vi "Main.vi"(8 "error in (no error)":errorcluster, 11 "RSABase in":refnum<class "RSA.lvclass">) -> (0 "error out":errorcluster, 3 "component":refnum<class "RSA.lvclass">)   [LabVIEW 2012, in "RSA.lvclass"]
doc: "Main VI of the component."
uses:
  RSA.lvclass
  <vilib>/Distrio/Murmex/Murmex/command_enum.ctl
  starting shape.ctl
  RSA.lvclass/RSA.ctl
  <vilib>/Distrio/Murmex/InitialiseMessage/InitialiseMessage.lvclass
  <vilib>/Distrio/Murmex/TerminateMessage/TerminateMessage.lvclass
  <vilib>/Distrio/Murmex/ConfigureMessage/ConfigureMessage.lvclass
  <vilib>/Distrio/Murmex/StartMessage/StartMessage.lvclass
  <vilib>/Distrio/Murmex/Murmex/update_cluster.ctl
  <vilib>/Distrio/Murmex/ResetMessage/ResetMessage.lvclass
  <vilib>/Distrio/Murmex/Murmex/Set configure at initialise.vi
  <vilib>/Distrio/Murmex/Murmex/Set log reference.vi
  <vilib>/Distrio/Murmex/Murmex/Set VI reference.vi
  <vilib>/Distrio/Murmex/Murmex/Get ID.vi
  <vilib>/Distrio/Murmex/Murmex/Murmex.lvclass
  <vilib>/Distrio/Murmex/Message/Message.lvclass
panel:
  in  "button::stop":bool
  in  "button::reset":bool
  in  "button::start":bool
  in  "button::quit":bool
  in  "Tab Control":enum32{"Settings", "Indicators", "Debug"}(tab)
  in  "Starting shape":T1
  in  "Bunch for averaging":i32=12
  in  "Wait time [ms]":u32=50
  in  "stop after":i32=500
  in  "Iterations until BC":i32=5000
  in  "Search Range [%]":dbl(knob)=100.0 min=0.0 max=100.0 step=5.0 scale=0.0..100.0
  in  "Optimisation name":string="bob"
  out "current MF":cluster{"Y":dbl[], "Y":dbl[]}[](graph)
  out "unsuccessfull iterations":i32
  out "successfull iterations":i32
  out "current Merit Factor":dbl
  out "Iterations since last improvement":i32
  out "max Merit Factor":dbl
  out "BC on":bool
  out "MF standard deviation":dbl
  out "best MF":cluster{"Y":dbl[], "Y":dbl[]}[](graph)
  out "BC counter":i32
  out "log":string="\r\n11:11:41.970 05/12/2013: initialise from AOTF to AOTF\r\n11:11:42.586 05/12/2013: inform from AOTF to AOTF\r\n11:11:43.913 05/12/2013: update from AOTF to AOTF\r\n11:11:45.142 05/12/2013: generic (shutter_off) from AOTF to AOTF\r\n11:11:45.270 05/12/2013: generic (shutter_on) from AOTF to AOTF\r\n11:11:45.902 05/12/2013: generic (shutter_off) from AOTF to AOTF\r\n11:11:45.932 05/12/2013: inspect from AOTF to AOTF\r\n11:11:48.013 05/12/2013: configure from AOTF to AOTF\r\n11:11:52.003 05/12/2013: inform from AOTF to AOTF\r\n11:11:58.521 05/12/2013: initialise from AOTF to AOTF\r\n11:11:58.561 05/12/2013: inform from AOTF to AOTF\r\n11:11:58.695 05/12/2013: inform from AOTF to AOTF\r\n11:12:02.089 05/12/2013: update from AOTF to AOTF\r\n11:12:02.308 05/12/2013: inspect from AOTF to AOTF\r\n11:12:02.364 05/12/2013: inform from AOTF to AOTF\r\n11:12:05.062 05/12/2013: generic (shutter_on) from AOTF to AOTF\r\n11:12:06.690 05/12/2013: update from AOTF to AOTF\r\n11:12:06.909 05/12/2013: inspect from AOTF to AOTF\r\n11:12:06.964 05/12/2013: inform from AOTF to AOTF\r\n11:12:07.770 05/12/2013: update from AOTF to AOTF\r\n11:12:07.989 05/12/2013: inspect from AOTF to AOTF\r\n11:12:08.044 05/12/2013: inform from AOTF to AOTF\r\n11:12:08.627 05/12/2013: update from AOTF to AOTF\r\n11:12:08.846 05/12/2013: inspect from AOTF to AOTF\r\n11:12:08.900 05/12/2013: inform from AOTF to AOTF\r\n11:12:09.290 05/12/2013: update from AOTF to AOTF\r\n11:12:09.508 05/12/2013: inspect from AOTF to AOTF\r\n11:12:09.563 05/12/2013: inform from AOTF to AOTF\r\n11:12:10.154 05/12/2013: update from AOTF to AOTF\r\n11:12:10.373 05/12/2013: inspect from AOTF to AOTF\r\n11:12:10.430 05/12/2013: inform from AOTF to AOTF\r\n11:12:20.953 05/12/2013: update from AOTF to AOTF\r\n11:12:21.172 05/12/2013: inspect from AOTF to AOTF\r\n11:12:21.227 05/12/2013: inform from AOTF to AOTF\r\n11:12:22.057 05/12/2013: update from AOTF to AOTF\r\n11:12:22.276 05/12/2013: inspect from AOTF to AOTF\r\n11:12:22.330 05/12/2013: inform from AOTF to AOTF\r\n11:12:22.841 05/12/2013: update from AOTF to AOTF\r\n11:12:23.060 05/12/2013: inspect from AOTF to AOTF\r\n11:12:23.114 05/12/2013: inform from AOTF to AOTF\r\n11:12:23.449 05/12/2013: update from AOTF to AOTF\r\n11:12:23.668 05/12/2013: inspect from AOTF to AOTF\r\n11:12:23.724 05/12/2013: inform from AOTF to AOTF\r\n11:12:24.514 05/12/2013: update from AOTF to AOTF\r\n11:12:24.733 05/12/2013: inspect from AOTF to AOTF\r\n11:12:24.789 05/12/2013: inform from AOTF to AOTF\r\n11:12:25.098 05/12/2013: update from AOTF to AOTF\r\n11:12:25.317 05/12/2013: inspect from AOTF to AOTF\r\n11:12:25.371 05/12/2013: inform from AOTF to AOTF\r\n11:12:26.482 05/12/2013: update from AOTF to AOTF\r\n11:12:26.701 05/12/2013: inspect from AOTF to AOTF\r\n11:12:26.755 05/12/2013: inform from AOTF to AOTF\r\n11:12:27.154 05/12/2013: update from AOTF to AOTF\r\n11:12:27.373 05/12/2013: inspect from AOTF to AOTF\r\n11:12:27.428 05/12/2013: inform from AOTF to AOTF\r\n11:12:27.666 05/12/2013: update from AOTF to AOTF\r\n11:12:27.885 05/12/2013: inspect from AOTF to AOTF\r\n11:12:27.944 05/12/2013: inform from AOTF to AOTF\r\n11:12:33.380 05/12/2013: update from AOTF to AOTF\r\n11:12:33.484 05/12/2013: update from AOTF to AOTF\r\n11:12:33.603 05/12/2013: inspect from AOTF to AOTF\r\n11:12:33.611 05/12/2013: update from AOTF to AOTF\r\n11:12:33.684 05/12/2013: update from AOTF to AOTF\r\n11:12:33.740 05/12/2013: update from AOTF to AOTF\r\n11:12:33.827 05/12/2013: inspect from AOTF to AOTF\r\n11:12:33.835 05/12/2013: update from AOTF to AOTF\r\n11:12:33.897 05/12/2013: inform from AOTF to AOTF\r\n11:12:33.903 05/12/2013: update from AOTF to AOTF\r\n11:12:33.940 05/12/2013: update from AOTF to AOTF\r\n11:12:34.085 05/12/2013: update from AOTF to AOTF\r\n11:12:34.119 05/12/2013: inspect from AOTF to AOTF\r\n11:12:34.292 05/12/2013: update from AOTF to AOTF\r\n11:12:34.336 05/12/2013: inspect from AOTF to AOTF\r\n11:12:34.553 05/12/2013: inspect from AOTF to AOTF\r\n11:12:34.608 05/12/2013: inform from AOTF to AOTF\r\n11:12:34.739 05/12/2013: update from AOTF to AOTF\r\n11:12:34.771 05/12/2013: update from AOTF to AOTF\r\n11:12:34.826 05/12/2013: inspect from AOTF to AOTF\r\n11:12:34.834 05/12/2013: update from AOTF to AOTF\r\n11:12:34.867 05/12/2013: update from AOTF to AOTF\r\n11:12:34.931 05/12/2013: update from AOTF to AOTF\r\n11:12:34.979 05/12/2013: update from AOTF to AOTF\r\n11:12:35.003 05/12/2013: update from AOTF to AOTF\r\n11:12:35.027 05/12/2013: update from AOTF to AOTF\r\n11:12:35.041 05/12/2013: update from AOTF to AOTF\r\n11:12:35.051 05/12/2013: inspect from AOTF to AOTF\r\n11:12:35.066 05/12/2013: update from AOTF to AOTF\r\n11:12:35.116 05/12/2013: update from AOTF to AOTF\r\n11:12:35.171 05/12/2013: update from AOTF to AOTF\r\n11:12:35.211 05/12/2013: update from AOTF to AOTF\r\n11:12:35.273 05/12/2013: inspect from AOTF to AOTF\r\n11:12:35.287 05/12/2013: update from AOTF to AOTF\r\n11:12:35.475 05/12/2013: update from AOTF to AOTF\r\n11:12:35.495 05/12/2013: inspect from AOTF to AOTF\r\n11:12:35.549 05/12/2013: inform from AOTF to AOTF\r\n11:12:35.764 05/12/2013: inspect from AOTF to AOTF\r\n11:12:35.819 05/12/2013: inform from AOTF to AOTF\r\n11:12:35.861 05/12/2013: update from AOTF to AOTF\r\n11:12:35.877 05/12/2013: inform from AOTF to AOTF\r\n11:12:35.947 05/12/2013: update from AOTF to AOTF\r\n11:12:36.067 05/12/2013: update from AOTF to AOTF\r\n11:12:36.100 05/12/2013: inspect from AOTF to AOTF\r\n11:12:36.235 05/12/2013: update from AOTF to AOTF\r\n11:12:36.317 05/12/2013: inspect from AOTF to AOTF\r\n11:12:36.371 05/12/2013: inform from AOTF to AOTF\r\n11:12:36.587 05/12/2013: inspect from AOTF to AOTF\r\n11:12:36.771 05/12/2013: update from AOTF to AOTF\r\n11:12:36.804 05/12/2013: inspect from AOTF to AOTF\r\n11:12:37.020 05/12/2013: inspect from AOTF to AOTF\r\n11:12:37.238 05/12/2013: inspect from AOTF to AOTF\r\n11:12:37.456 05/12/2013: inspect from AOTF to AOTF\r\n11:12:37.673 05/12/2013: inspect from AOTF to AOTF\r\n11:12:37.891 05/12/2013: inspect from AOTF to AOTF\r\n11:12:37.946 05/12/2013: inform from AOTF to AOTF\r\n11:12:38.161 05/12/2013: inspect from AOTF to AOTF\r\n11:12:38.379 05/12/2013: inspect from AOTF to AOTF\r\n11:12:38.597 05/12/2013: inspect from AOTF to AOTF\r\n11:12:38.815 05/12/2013: inspect from AOTF to AOTF\r\n11:12:38.871 05/12/2013: inform from AOTF to AOTF\r\n11:12:39.086 05/12/2013: inspect from AOTF to AOTF\r\n11:12:39.303 05/12/2013: inspect from AOTF to AOTF\r\n11:12:39.363 05/12/2013: inform from AOTF to AOTF\r\n11:12:39.417 05/12/2013: inform from AOTF to AOTF\r\n11:12:39.633 05/12/2013: inspect from AOTF to AOTF\r\n11:12:39.852 05/12/2013: inspect from AOTF to AOTF\r\n11:12:40.069 05/12/2013: inspect from AOTF to AOTF\r\n11:12:40.124 05/12/2013: inform from AOTF to AOTF\r\n11:12:40.339 05/12/2013: inspect from AOTF to AOTF\r\n11:12:40.395 05/12/2013: inform from AOTF to AOTF\r\n11:12:40.448 05/12/2013: inform from AOTF to AOTF\r\n11:12:40.663 05/12/2013: inspect from AOTF to AOTF\r\n11:12:40.718 05/12/2013: inform from AOTF to AOTF\r\n11:12:40.770 05/12/2013: inform from AOTF to AOTF\r\n11:12:40.824 05/12/2013: inform from AOTF to AOTF\r\n11:12:40.877 05/12/2013: inform from AOTF to AOTF\r\n11:12:40.930 05/12/2013: inform from AOTF to AOTF\r\n11:12:40.982 05/12/2013: inform from AOTF to AOTF\r\n11:12:41.034 05/12/2013: inform from AOTF to AOTF\r\n11:12:41.092 05/12/2013: inform from AOTF to AOTF\r\n11:12:41.144 05/12/2013: inform from AOTF to AOTF\r\n11:12:41.196 05/12/2013: inform from AOTF to AOTF\r\n11:12:41.249 05/12/2013: inform from AOTF to AOTF\r\n11:12:41.307 05/12/2013: inform from AOTF to AOTF\r\n11:12:41.366 05/12/2013: inform from AOTF to AOTF\r\n11:12:41.424 05/12/2013: inform from AOTF to AOTF\r\n11:12:41.478 05/12/2013: inform from AOTF to AOTF\r\n11:12:41.533 05/12/2013: inform from AOTF to AOTF\r\n11:12:41.589 05/12/2013: inform from AOTF to AOTF\r\n11:12:42.246 05/12/2013: terminate from AOTF to AOTF"
  in  "component ID":string="RSA"
  in  "command":T2
  in  "Generic command":string
  in  "button::configure":bool
  in  "button::send":bool
  out "terminate?":bool=TRUE
  # "RSA settings"
  # "Save settings"
  # "Bleaching compensation"
  # "Iterations"
  # "Merit Factor"
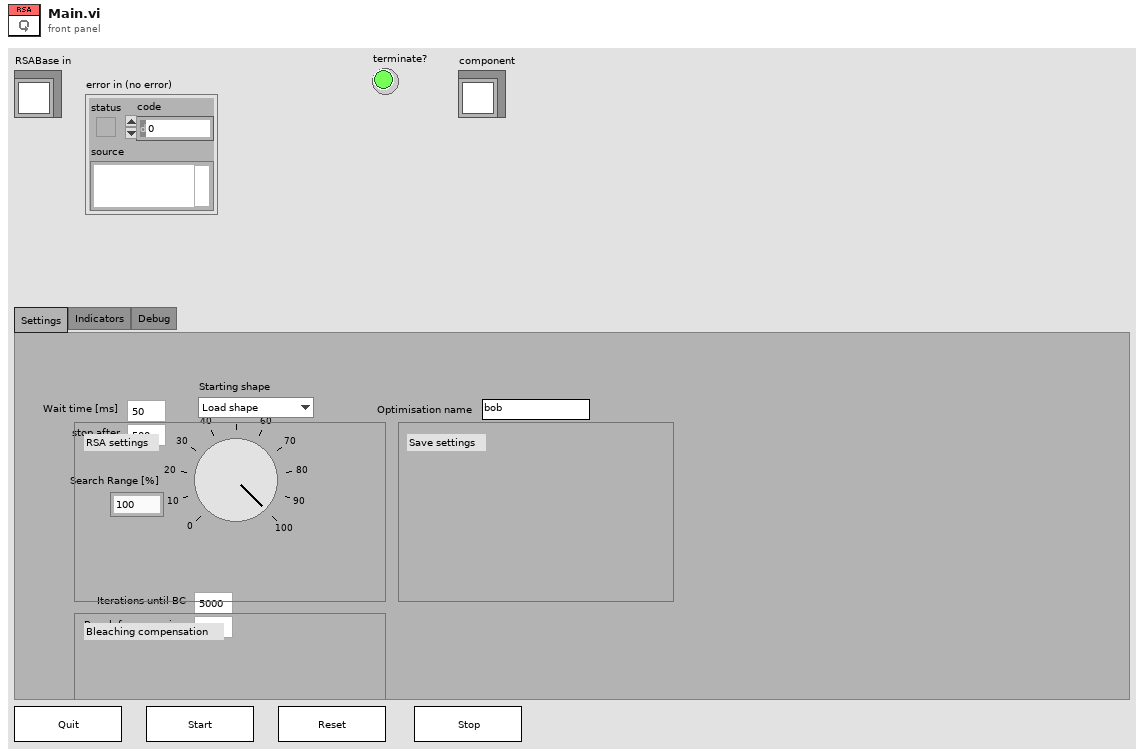
[diagram p1: front panel]
types:
  T1 = typedef "RSA.lvclass/starting shape.ctl" = enum16{"Load shape", "Midrange"}
  T2 = typedef "Murmex.lvlib/Murmex.lvclass/command_enum.ctl" = enum16{"null", "initialise", "reset", "terminate", "acknowledge", "update", "inspect", "inform", "proceed", "start", "stop", "fetch", "configure", "generic"}
  T3 = typedef "Murmex.lvlib/Murmex.lvclass/update_cluster.ctl" = cluster{"target ID":string, "key chains":string[], "values":variant[]}
  T4 = enum8{"Enabled", "Disabled", "Disabled and Grayed Out"}
  T5 = typedef "Murmex.lvclass/command_enum.ctl" = enum16{"null", "initialise", "reset", "terminate", "acknowledge", "update", "inspect", "inform", "proceed", "start", "stop", "fetch", "configure", "generic"}
  T6 = typedef "Murmex.lvclass/Event type enumerations.ctl" = enum16{"before", "after"}
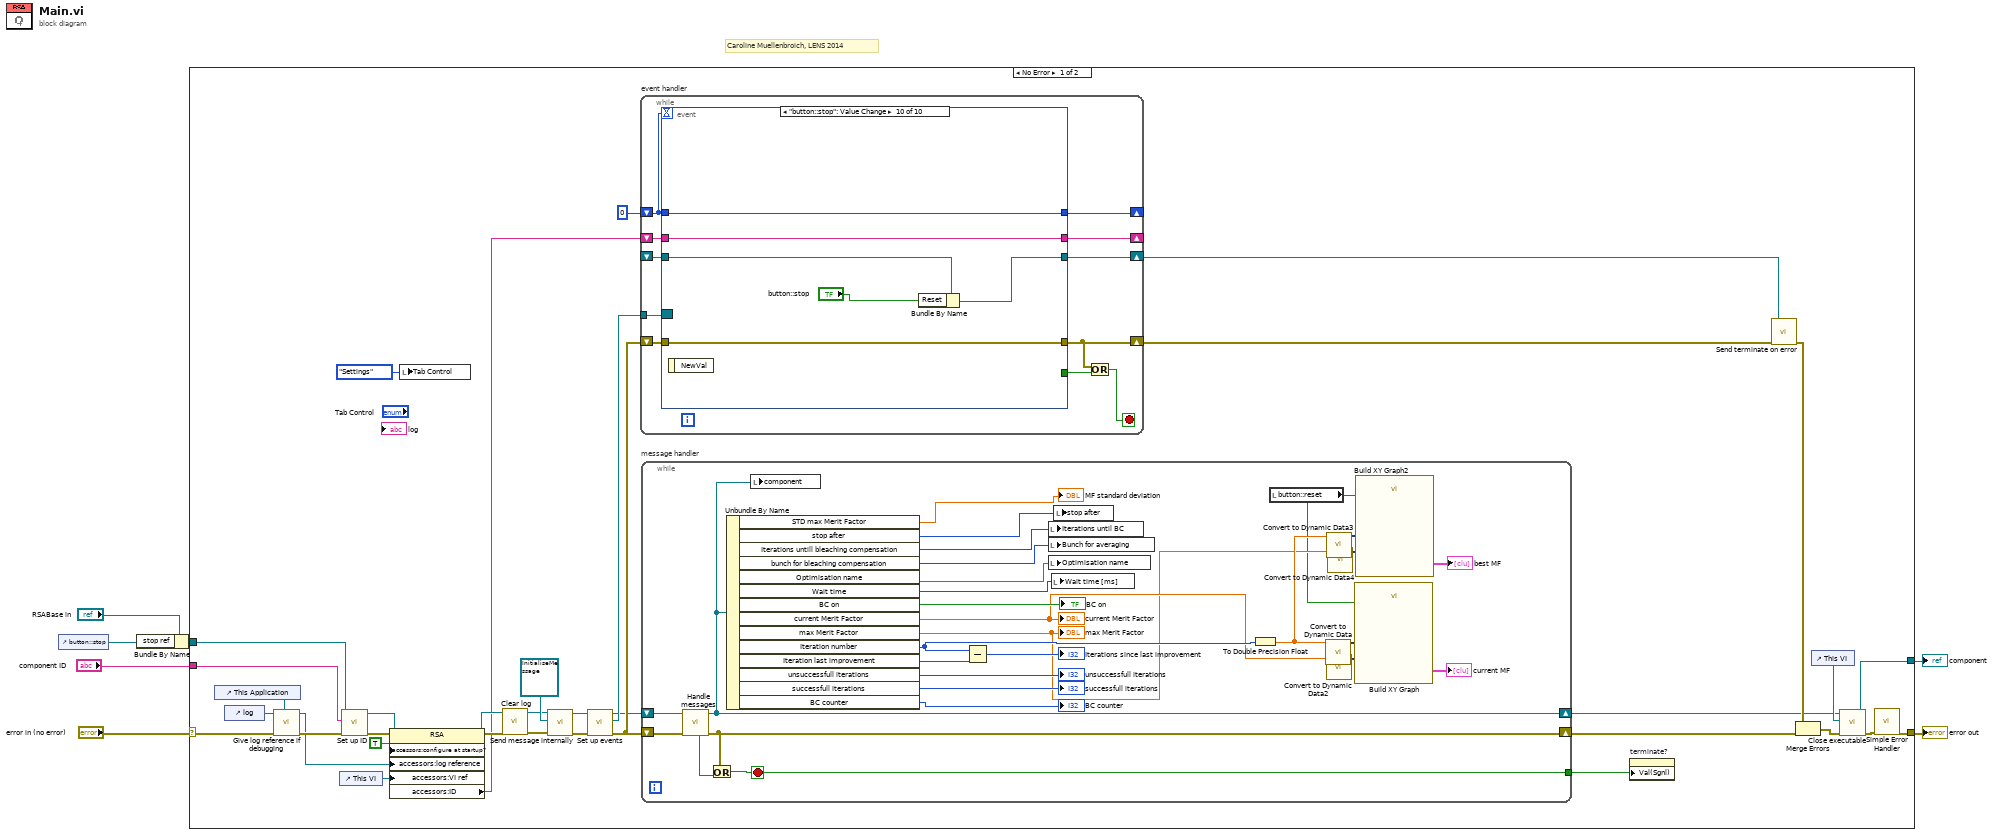
[diagram p0: block diagram]
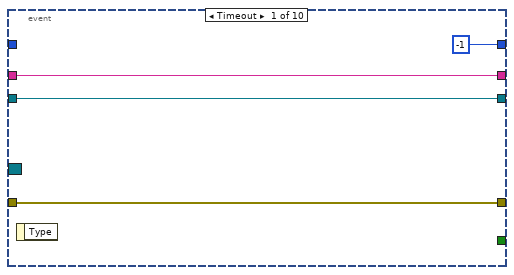
[diagram p2: hidden frame]
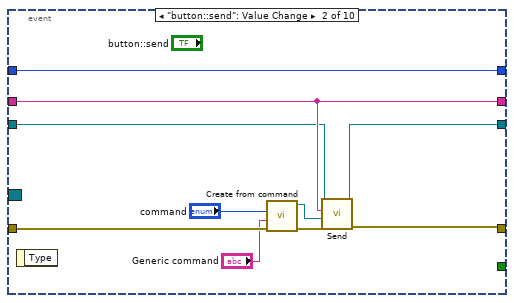
[diagram p3: hidden frame]
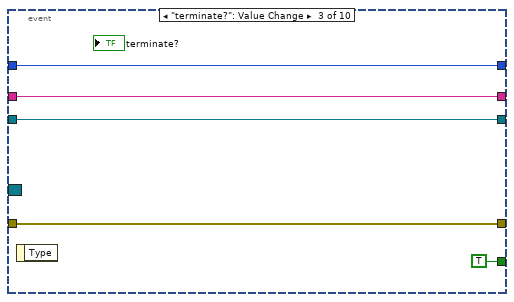
[diagram p4: hidden frame]
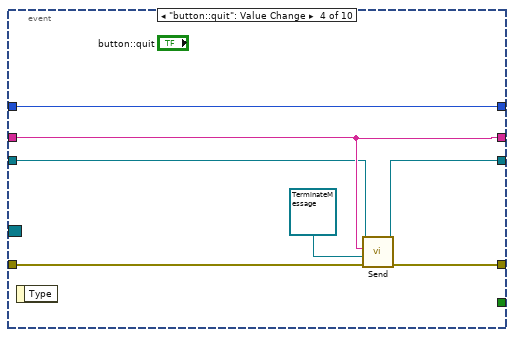
[diagram p5: hidden frame]
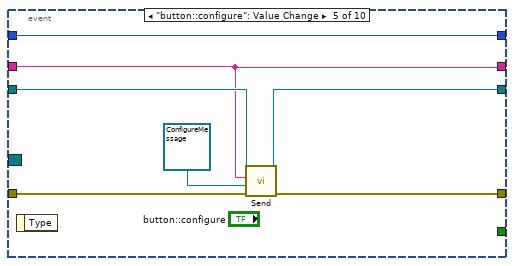
[diagram p6: hidden frame]
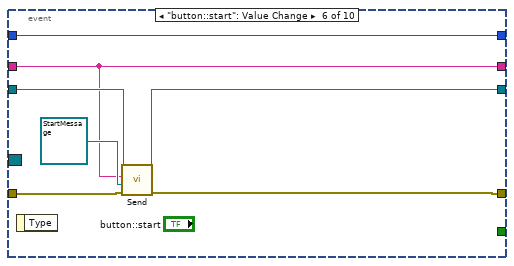
[diagram p7: hidden frame]
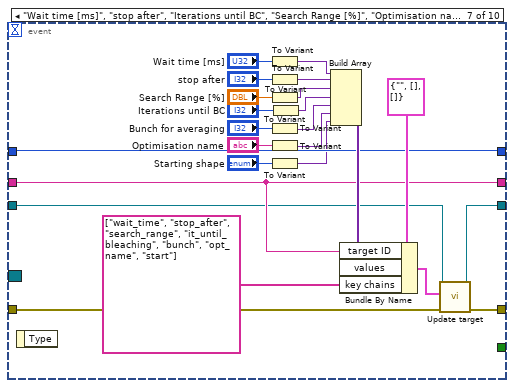
[diagram p8: hidden frame]
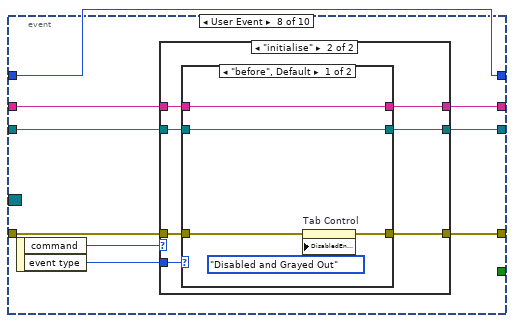
[diagram p9: hidden frame]
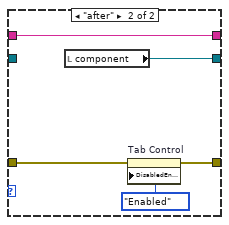
[diagram p11: hidden frame]
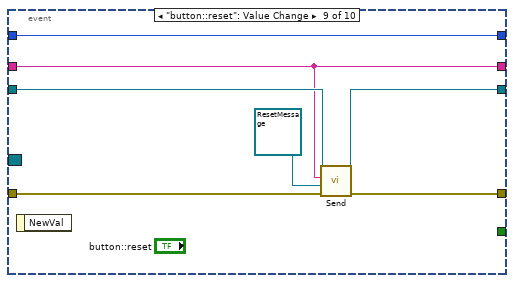
[diagram p12: hidden frame]
diagram:
  # "Caroline Muellenbroich, LENS 2014"
  n1 = control-ref of="button::stop"() -> (w3:refnum<vi>)
  n2 = Bundle By Name(cluster="RSABase in", "stop ref"=w3) -> (w1:refnum<class "RSA.lvclass">)
  n3 = case shown="No Error" "error in (no error)" {
    selector: "error in (no error)" -> [w12 w190]
    tunnel: w1 -> [w38 w189]
    tunnel: "component ID" -> [w37 _]
    tunnel: [w18 w189] -> w5
    tunnel: [w16 w190] -> w4
    frame No Error {
      n4 = control-ref of="This Application"() -> (w8:refnum<vi>)
      n5 = control-ref of="log"() -> (w10:refnum<vi>)
      n6 = call "Give log reference if debugging.vi"("application ref"=w8, "error in (no error)"=w12, "log reference in"=w10) -> ("error out"=w11:errorcluster, "log reference out"=w9:refnum<vi>)  [unwired: 6 in, 1 out]
      n7 = control-ref of="This VI"() -> (w42:refnum<vi>)
      n8 = call <vilib>:"Set up ID.vi"("error in (no error)"=w11, "component ID"=w37, "MurmexBase in"=w38) -> ("error out"=w39:errorcluster, "MurmexBase out"=w40:refnum<class "RSA.lvclass">)  [unwired: 6 in, 1 out]
      n9 = property class="RSA"(reference=w40, error in=w39, "accessors:configure at startup?"=TRUE ("configure at startup?"), "accessors:log reference"=w9, "accessors:VI ref"=w42) -> (reference out=w30:refnum<class "RSA.lvclass">, error out=w31:errorcluster, "accessors:ID"=w29:string)
      n10 = local write "Tab Control"(enum32{"Settings", "Indicators", "Debug"}."Settings" ("Tab Control")) -> ()
      n11 = call <vilib>:"Clear log.vi"("error in (no error)"=w31, "MurmexBase in"=w30) -> ("error out"=w32:errorcluster, "MurmexBase out"=w33:refnum<class "RSA.lvclass">)  [unwired: 8 in]
      n12 = call <vilib>:"Send message internally.vi"("error in (no error)"=w32, "Message"=refnum<class "InitialiseMessage.lvclass"> refnum ("Murmex.lvlib:InitialiseMessage"), "Murmex in"=w33) -> ("error out"=w34:errorcluster, "Murmex out"=w35:refnum<class "RSA.lvclass">)  [unwired: 7 in]
      n13 = call <vilib>:"Set up events.vi"("error in (no error)"=w34, "MurmexBase in"=w35) -> ("error out"=w27:errorcluster, "Event Registration Refnum"=w28:refnum<event-registration>, "MurmexBase out"=w26:refnum<class "RSA.lvclass">)  [unwired: 7 in]
      n14 = while "event handler" {
        shift-right: [w78] -> _
        shift-left: w29 -> [w81]
        shift-right: [w77] -> w24
        shift-left: w27 -> [w82]
        shift-right: [w79] -> _
        shift-left: 0 -> [w80]
        shift-right: [w74] -> w15
        shift-left: _ -> [w73]
        tunnel: w28 -> [w75]
        stop <- w76 stop-if-true
        n15 = event shown="[9] \"button::stop\": Value Change" {
          selector: w75 -> [_ _ _ _ _ _ _ _ _ _]
          dyn-events: _ -> [_ _ _ _ _ _ _ _ _ _]
          timeout: w80 -> [_ _ _ _ _ _ _ _ _ _]
          tunnel: w82 -> [w84 w94 w97 w107 w114 w122 w146 w150 w182 w186]
          tunnel: w81 -> [w85 w90 w99 w105 w110 w117 w135 w153 w177 w187]
          tunnel: w80 -> [_ w87 w100 w102 w109 w116 w134 w151 w176 w188]
          tunnel: [-1 w87 w100 w102 w109 w116 w134 w151 w176 w188] -> w79
          tunnel: [w85 w90 w99 w105 w110 w117 w135 w152 w177 w187] -> w78
          tunnel: [w84 w93 w97 w106 w113 w121 w145 w149 w181 w186] -> w77
          tunnel: [w83 w88 w98 w103 w111 w118 w139 w148 w178 w184] -> w74
          tunnel: w73 -> [w83 w89 w98 w104 w112 w119 w126 w147 w179 w185]
          tunnel: [_ _ TRUE _ _ _ _ _ _ _] -> w72
          event Timeout {
            n16 = event-data() -> ()  [unwired: 1 in, 1 out]
          }
          event "button::send": Value Change {
            n17 = event-data() -> ()  [unwired: 1 in, 1 out]
            n18 = call <vilib>:"Create from command.vi"("error in (no error)"=w94, "generic command"="Generic command", "command"="command") -> ("error out"=w95:errorcluster, "Message out"=w96:refnum<class "Message.lvclass">)  [unwired: 7 in]
            n19 = call <vilib>:"Send.vi"("error in (no error)"=w95, "Message"=w96, "recipient"=w90, "Murmex in"=w89) -> ("error out"=w93:errorcluster, "Murmex out"=w88:refnum<class "RSA.lvclass">)  [unwired: 6 in]
          }
          event "terminate?": Value Change {
            n20 = event-data() -> ()  [unwired: 1 in, 1 out]
          }
          event "button::quit": Value Change {
            n21 = event-data() -> ()  [unwired: 1 in, 1 out]
            n22 = call <vilib>:"Send.vi"("error in (no error)"=w107, "Message"=refnum<class "TerminateMessage.lvclass"> refnum ("Murmex.lvlib:TerminateMessage"), "recipient"=w105, "Murmex in"=w104) -> ("error out"=w106:errorcluster, "Murmex out"=w103:refnum<class "RSA.lvclass">)  [unwired: 6 in]
          }
          event "button::configure": Value Change {
            n23 = event-data() -> ()  [unwired: 1 in, 1 out]
            n24 = call <vilib>:"Send.vi"("error in (no error)"=w114, "Message"=refnum<class "ConfigureMessage.lvclass"> refnum ("Murmex.lvlib:ConfigureMessage"), "recipient"=w110, "Murmex in"=w112) -> ("error out"=w113:errorcluster, "Murmex out"=w111:refnum<class "RSA.lvclass">)  [unwired: 6 in]
          }
          event "button::start": Value Change {
            n25 = event-data() -> ()  [unwired: 1 in, 1 out]
            n26 = call <vilib>:"Send.vi"("error in (no error)"=w122, "Message"=refnum<class "StartMessage.lvclass"> refnum ("Message in"), "recipient"=w117, "Murmex in"=w119) -> ("error out"=w121:errorcluster, "Murmex out"=w118:refnum<class "RSA.lvclass">)  [unwired: 6 in]
          }
          event "Wait time [ms]", "stop after", "Iterations until BC", "Search Range [%]", "Optimisation name", "Bunch for averaging": Value Change {
            n27 = event-data() -> ()  [unwired: 1 in, 1 out]
            n28 = To Variant(anything="Wait time [ms]") -> (Variant=w141:variant)
            n29 = To Variant(anything="stop after") -> (Variant=w144:variant)
            n30 = To Variant(anything="Search Range [%]") -> (Variant=w143:variant)
            n31 = To Variant(anything="Bunch for averaging") -> (Variant=w128:variant)
            n32 = To Variant(anything="Optimisation name") -> (Variant=w129:variant)
            n33 = To Variant(anything="Starting shape") -> (Variant=w123:variant)
            n34 = To Variant(anything="Iterations until BC") -> (Variant=w142:variant)
            n35 = Build Array(w141, w144, w143, w142, w128, w129, w123) -> (w138:variant[])
            n36 = Bundle By Name(cluster=T3 {"target ID"="", "key chains"=[], "values"=[]} ("update cluster"), "target ID"=w135, "values"=w138, "key chains"=string[] ["wait_time", "stop_after", "search_range", "it_until_bleaching", "bunch", "opt_name", "start"]) -> (w140:T3)
            n37 = call <vilib>:"Update target.vi"("error in (no error)"=w146, "update cluster"=w140, "MurmexBase in"=w126) -> ("error out"=w145:errorcluster, "MurmexBase out"=w139:refnum<class "RSA.lvclass">)  [unwired: 7 in]
          }
          event User Event {
            n38 = event-data() -> ("command"=w155:T5, "event type"=w154:T6)  [unwired: 1 in]
            n39 = case shown="\"initialise\"" w155 {
              tunnel: w154 -> [_ w165]
              tunnel: w153 -> [w158 w164]
              tunnel: [w158 w163] -> w152
              tunnel: w150 -> [w157 w162]
              tunnel: [w157 w161] -> w149
              tunnel: [w156 w160] -> w148
              tunnel: w147 -> [w156 w159]
              frame "null", Default {
              }
              frame "initialise" {
                n40 = case shown="\"before\", Default" w165 {
                  tunnel: w164 -> [w170 w175]
                  tunnel: [w170 w175] -> w163
                  tunnel: w162 -> [w167 w173]
                  tunnel: [w166 w172] -> w161
                  tunnel: [w169 w174] -> w160
                  tunnel: w159 -> [w169 _]
                  frame "before", Default {
                    n41 = property on="Tab Control" class="TabCtl (strict)"(error in=w167, "DisabledEnum"=T4."Disabled and Grayed Out" ("Disabled")) -> (error out=w166:errorcluster)  [unwired: 1 in, 1 out]
                  }
                  frame "after" {
                    n42 = local read "component"() -> (w174:refnum<class "RSA.lvclass">)
                    n43 = property on="Tab Control" class="TabCtl (strict)"(error in=w173, "DisabledEnum"=T4."Enabled" ("Disabled")) -> (error out=w172:errorcluster)  [unwired: 1 in, 1 out]
                  }
                }
              }
            }
          }
          event "button::reset": Value Change {
            n44 = event-data() -> ()  [unwired: 1 in, 1 out]
            n45 = call <vilib>:"Send.vi"("error in (no error)"=w182, "Message"=refnum<class "ResetMessage.lvclass"> refnum ("Distrio Murmex 1.0:ResetMessage"), "recipient"=w177, "Murmex in"=w179) -> ("error out"=w181:errorcluster, "Murmex out"=w178:refnum<class "RSA.lvclass">)  [unwired: 6 in]
          }
          event "button::stop": Value Change {
            n46 = event-data() -> ()  [unwired: 1 in, 1 out]
            n47 = Bundle By Name(cluster=w185, "Reset"="button::stop") -> (w184:refnum<class "RSA.lvclass">)
          }
        }
        n48 = Or(x=w77, y=w72) -> (x .or. y?=w76:bool)
      }
      n49 = while "message handler" {
        shift-right: [w68] -> w23
        shift-left: w27 -> [w70]
        shift-right: [w51] -> w19
        shift-left: w26 -> [w69]
        tunnel: [w67] -> w13
        stop <- w67 stop-if-true
        n50 = call <vilib>:"Handle messages.vi"("error in (no error)"=w70, "Murmex in"=w69) -> ("error out"=w68:errorcluster, "Murmex out"=w51:refnum<class "RSA.lvclass">, "terminated?"=w71:bool)  [unwired: 7 in]
        n51 = Or(x=w68, y=w71) -> (x .or. y?=w67:bool)
        n52 = Unbundle By Name(w51) -> ("STD max Merit Factor"=→"MF standard deviation":dbl, "stop after"=w53:i32, "Iterations untill bleaching compensation"=w52:i32, "bunch for bleaching compensation"=w54:i32, "Optimisation name"=w55:string, "Wait time"=w56:u32, "BC on"=→"BC on":bool, "current Merit Factor"=w57:dbl, "max Merit Factor"=w45:dbl, "Iteration number"=w60:i32, "Iteration last improvement"=w66:i32, "unsuccessfull iterations"=→"unsuccessfull iterations":i32, "successfull iterations"=→"successfull iterations":i32, "BC counter"=→"BC counter":i32)
        "current Merit Factor" <- w57
        "max Merit Factor" <- w45
        n53 = local write "component"(w51) -> ()
        n54 = Subtract(x=w60, y=w66) -> (x-y=→"Iterations since last improvement":i32)
        n55 = local write "Iterations until BC"(w52) -> ()
        n56 = local write "Bunch for averaging"(w54) -> ()
        n57 = local write "Optimisation name"(w55) -> ()
        n58 = local write "Wait time [ms]"(w56) -> ()
        n59 = local write "stop after"(w53) -> ()
        n60 = To Double Precision Float(number=w60) -> (double precision float=w47:dbl)
        n61 = local read "button::reset"() -> (w44:bool)
        n62 = call "Convert to Dynamic Data"("Double"=w47) -> ("Dynamic Data Type"=w59:dynamicdata)  [unwired: 3 in]
        n63 = call "Convert to Dynamic Data3"("Double"=w47) -> ("Dynamic Data Type"=w49:dynamicdata)  [unwired: 3 in]
        n64 = call "Convert to Dynamic Data2"("Double"=w57) -> ("Dynamic Data Type"=w58:dynamicdata)  [unwired: 3 in]
        n65 = call "Convert to Dynamic Data4"("Double"=w45) -> ("Dynamic Data Type"=w50:dynamicdata)  [unwired: 3 in]
        n66 = call "Build XY Graph"("Reset"=w44, "Y Input"=w58, "X Input"=w59) -> ("XY Graph"=→"current MF":cluster{"Y":dbl[], "Y":dbl[]}[])  [unwired: 2 in, 6 out]
        n67 = call "Build XY Graph2"("Reset"=w44, "Y Input"=w50, "X Input"=w49) -> ("XY Graph"=→"best MF":cluster{"Y":dbl[], "Y":dbl[]}[])  [unwired: 2 in, 6 out]
      }
      n68 = property on="terminate?" class="Bool (strict)"("Val(Sgnl)"=w13) -> ()  [unwired: 2 in, 2 out]
      n69 = call <vilib>:"Send terminate on error.vi"("error in (no error)"=w24, "Murmex in"=w15) -> ("error out"=w22:errorcluster)  [unwired: 8 in, 1 out]
      n70 = Merge Errors(w22, w23) -> (w21:errorcluster)
      n71 = control-ref of="This VI"() -> (w20:refnum<vi>)
      n72 = call <vilib>:"Close executable.vi"("error in (no error)"=w21, "main VI ref (optional)"=w20, "MurmexBase in"=w19) -> ("error out"=w17:errorcluster, "MurmexBase out"=w18:refnum<class "RSA.lvclass">)  [unwired: 7 in]
      n73 = call <vilib>:"Simple Error Handler.vi"("error in (no error)"=w17) -> ("error out"=w16:errorcluster)  [unwired: 4 in, 4 out]
    }
    frame Error {
    }
  }
  "error out" <- w4
  "component" <- w5
